vi "i64_to_fxpe.vi"(1 "64bit integer":i64) -> (0 "fxp64_32":fxp<+/-,64,32>)   [LabVIEW 2018]
uses:
  <vilib>/rvi/FXPMathLib/FxpInterpret/XNode/nifxpmath_Interpret.xnode
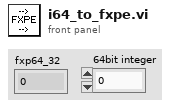
[diagram p1: front panel]
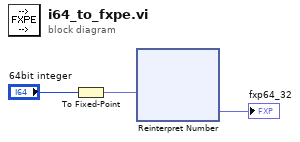
[diagram p0: block diagram]
diagram:
  n1 = To Fixed-Point(number="64bit integer") -> (fixed-point=w3:fxp<+/-,64,64>)  [unwired: 1 in]
  n2 = xnode "Reinterpret Number"("x"=w3) -> ("y"=→"fxp64_32":fxp<+/-,64,32>)
